vi "Config_LoadKeys.vi"(8 "error in (no error)":errorcluster, 11 "Config In":T3) -> (0 "error out":errorcluster, 2 "output cluster":T1={"General"={"Config.ini"=path "", "Default Logging Path"=path ""}, "Hardware"={"AHC VISA COM"="", "Measure Rate (1/s)"=0, "Global T VAR"="", "Global B VAR"=""}, "Operation"={"Operation Mode"=enum."Idle-Off", "Status"="", "NewLog?"=FALSE}}, 3 "refnum out":T3)   [LabVIEW 2021]
uses:
  <vilib>/Utility/config.llb/Config Data RefNum.ctl
  Config_Cluster.ctl
  Mode_Enum.ctl
  <vilib>/Utility/config.llb/Read Key (Path).vi
  <vilib>/Utility/config.llb/Read Key (String).vi
  <vilib>/Utility/config.llb/Read Key (I32).vi
  <vilib>/Utility/config.llb/NI_LVConfig.lvlib
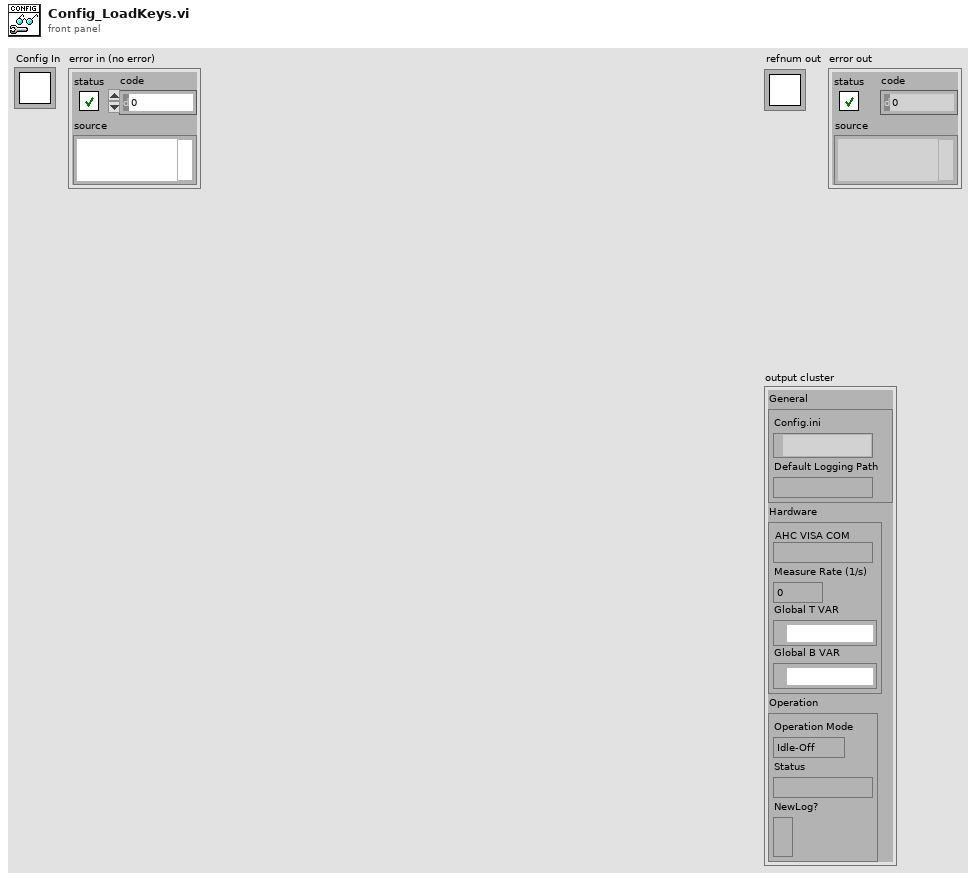
[diagram p1: front panel]
types:
  T1 = typedef "Config_Cluster.ctl" = cluster{"General":cluster{"Config.ini":path, "Default Logging Path":path}, "Hardware":cluster{"AHC VISA COM":refnum<visa-resource-name>, "Measure Rate (1/s)":i32, "Global T VAR":refnum<k21>, "Global B VAR":refnum<k21>}, "Operation":cluster{"Operation Mode":T2, "Status":string, "NewLog?":bool}}
  T2 = typedef "Mode_Enum.ctl" = enum16{"Logging", "Idle-Off", "Idle"}
  T3 = typedef "NI_LVConfig.lvlib/Config Data RefNum.ctl" = refnum<k1>
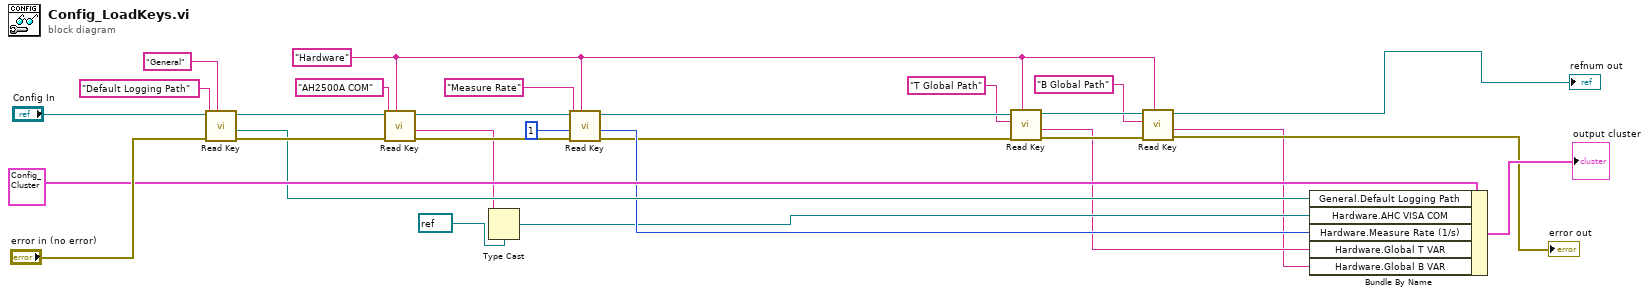
[diagram p0: block diagram]
diagram:
  w8 = "Hardware" ("section")
  n1 = call-poly <vilib>:"Read Key.vi"("section"="General", "error in (no error)"="error in (no error)", "key"="Default Logging Path", "refnum"="Config In") -> ("error out"=w23:errorcluster, "value"=w21:path, "refnum out"=w25:T3)  [unwired: 4 in, 1 out]
  n2 = call-poly <vilib>:"Read Key.vi"("section"=w8, "error in (no error)"=w23, "key"="AH2500A COM", "refnum"=w25) -> ("error out"=w18:errorcluster, "value"=w14:string, "refnum out"=w20:T3)  [unwired: 4 in, 1 out]
  n3 = Type Cast(type=refnum<visa-resource-name> refnum ("VISA resource name"), x=w14) -> (*(type *) &x=w16:refnum<visa-resource-name>)
  n4 = call-poly <vilib>:"Read Key.vi"("section"=w8, "error in (no error)"=w18, "default value"=1, "key"="Measure Rate", "refnum"=w20) -> ("error out"=w10:errorcluster, "value"=w17:i32, "refnum out"=w11:T3)  [unwired: 3 in, 1 out]
  n5 = call-poly <vilib>:"Read Key.vi"("section"=w8, "error in (no error)"=w10, "key"="T Global Path", "refnum"=w11) -> ("error out"=w6:errorcluster, "value"=w2:string, "refnum out"=w9:T3)  [unwired: 4 in, 1 out]
  n6 = call-poly <vilib>:"Read Key.vi"("section"=w8, "error in (no error)"=w6, "key"="B Global Path", "refnum"=w9) -> ("error out"=→"error out":errorcluster, "value"=w1:string, "refnum out"=→"refnum out":T3)  [unwired: 4 in, 1 out]
  n7 = Bundle By Name(cluster=T1 {"General"={"Config.ini"=path "", "Default Logging Path"=path ""}, "Hardware"={"AHC VISA COM"="", "Measure Rate (1/s)"=0, "Global T VAR"="", "Global B VAR"=""}, "Operation"={"Operation Mode"=enum."Logging", "Status"="", "NewLog?"=FALSE}} ("Configuration Cluster"), "General.Default Logging Path"=w21, "Hardware.AHC VISA COM"=w16, "Hardware.Measure Rate (1/s)"=w17, "Hardware.Global T VAR"=w2, "Hardware.Global B VAR"=w1) -> (→"output cluster":T1)
